vi "Initialize.vi"(0 "TCP Socket In":refnum<class "Socket Communication.lvclass">, 5 "error in (no error)":errorcluster) -> (14 "TCP Socket Out":refnum<class "Socket Communication.lvclass">, 19 "error out":errorcluster)   [LabVIEW 2016, in "Socket Communication.lvclass"]
uses:
  Socket Communication.lvclass
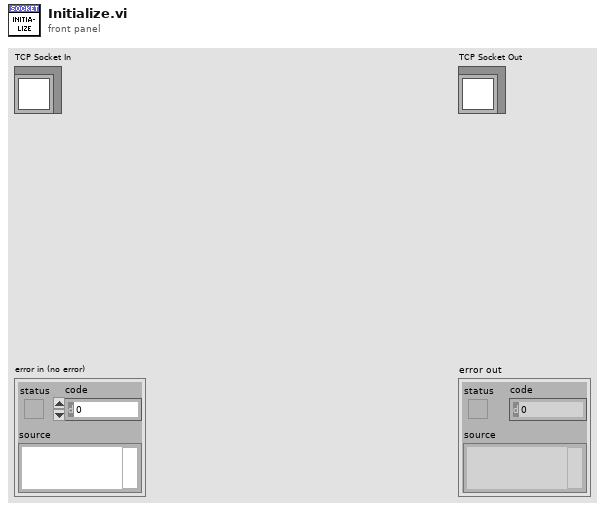
[diagram p1: front panel]
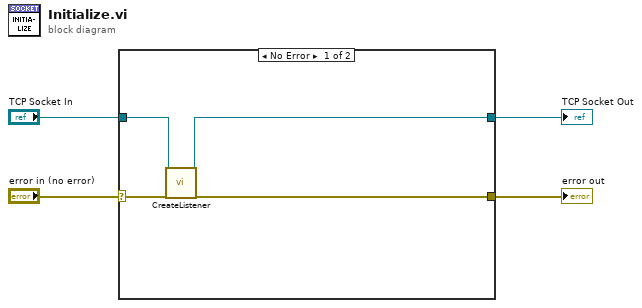
[diagram p0: block diagram]
diagram:
  n1 = case shown="No Error" "error in (no error)" {
    selector: "error in (no error)" -> [w8 w10]
    tunnel: [w6 w10] -> w4
    tunnel: [w5 w9] -> w3
    tunnel: "TCP Socket In" -> [w7 w9]
    frame No Error {
      n2 = call "CreateListener.vi"("Socket Listener in"=w7, "error in (no error)"=w8) -> ("Socket Listener out"=w5:refnum<class "Socket Communication.lvclass">, "error out"=w6:errorcluster)  [unwired: 16 in]
    }
    frame Error {
    }
  }
  "error out" <- w4
  "TCP Socket Out" <- w3
